vi "Construct Persist To Disk Transport.vi"(10 "Datum Name":string, 11 "Folder Path":path) -> (0 "error out":errorcluster, 3 "PersistToDiskTransport":refnum<class "PersistToDiskTransport.lvclass">)   [LabVIEW 2019, in "PersistToDiskTransport.lvclass"]
doc: "<License>\nCopyright © 2017 Composed Systems, LLC | All rights reserved\nwww.composed.io\n\nAuthor: Ethan Stern <ethan.stern@composed.io>\n\nThis software is provided \"AS IS\" WITHOUT WARRANTIES, either express or implied, AND IS FOR EDUCATIONAL PURPOSES ONLY.\n</License>"
uses:
  <vilib>/gpm_packages/@cs/transport/Source/Concrete/PersistToDiskTransport/PersistToDiskTransport.lvclass
  <vilib>/gpm_packages/@cs/transport/Source/Concrete/PersistToDiskTransport/PersistToDiskTransport.lvclass/PersistToDiskTransport.ctl
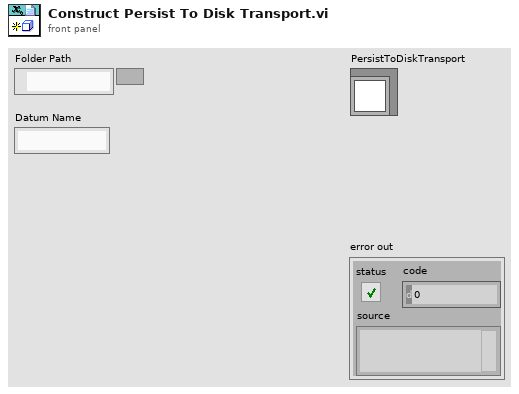
[diagram p1: front panel]
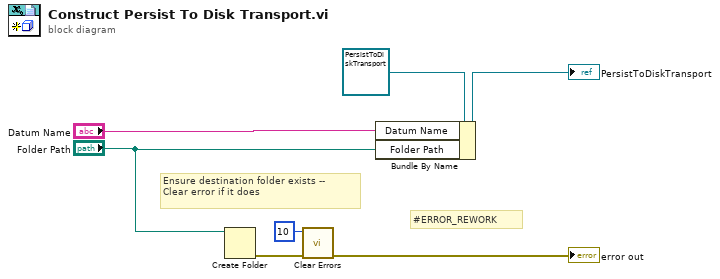
[diagram p0: block diagram]
diagram:
  # "#ERROR_REWORK"
  # "Ensure destination folder exists --\nClear error if it does"
  n1 = Create Folder(path (use dialog)="Folder Path") -> (error out=w5:errorcluster)  [unwired: 2 in, 2 out]
  n2 = call <vilib>:"Clear Errors.vi"("error in (no error)"=w5, "specific error code to clear (0: all)"=10) -> ("error out"=→"error out":errorcluster)  [unwired: 4 in, 1 out]
  n3 = Bundle By Name(cluster=refnum<class "PersistToDiskTransport.lvclass"> refnum ("PersistToDiskTransport"), "Datum Name"="Datum Name", "Folder Path"="Folder Path") -> (→"PersistToDiskTransport":refnum<class "PersistToDiskTransport.lvclass">)
